vi "Delete 1D array elements.vi"(9 "Elements to delete":i32[](array[numeric]), 11 "Input array":i32[](array[numeric])) -> (3 "Array w elements deleted":i32[](array[numeric]))   [LabVIEW 2017]
doc: "Searches for the specified elements and deletes them from the input array"
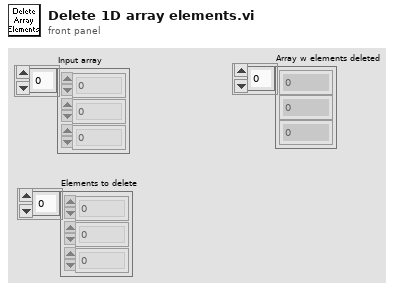
[diagram p1: front panel]
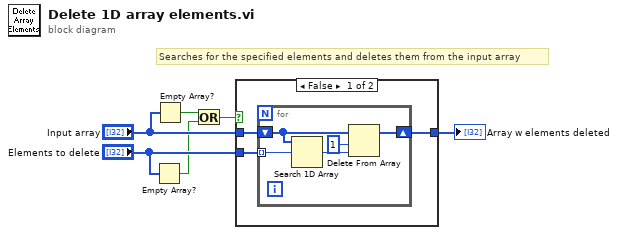
[diagram p0: block diagram]
diagram:
  # "Searches for the specified elements and deletes them from the input array"
  n1 = Empty Array?(array="Elements to delete") -> (empty?=w2:bool)
  n2 = Empty Array?(array="Input array") -> (empty?=w3:bool)
  n3 = Or(x=w3, y=w2) -> (x .or. y?=w1:bool)
  n4 = case shown="False" w1 {
    tunnel: [w9 w15] -> w6
    tunnel: "Input array" -> [w8 w15]
    tunnel: "Elements to delete" -> [w7 _]
    frame False {
      n5 = for {
        tunnel: w7 -> [w14] mode=indexing
        shift-right: [w10] -> w9
        shift-left: w8 -> [w12]
        n6 = Search 1D Array(1D array=w12, element=w14) -> (index of element=w13:i32)  [unwired: 1 in]
        n7 = Delete From Array(array=w12, length=1, index=w13) -> (array with subset deleted=w10:i32[])  [unwired: 1 out]
      }
    }
    frame True {
    }
  }
  "Array w elements deleted" <- w6
